vi "Autonomous Independent.vi"() -> ()   [LabVIEW 2019]
doc: "This VI is called when autonomous begins, and will automatically be terminated when autonomous ends. You can carry out timed or sensor driven robot movement independently without needing to return to the caller."
uses:
  <vilib>/Rock Robotics/WPI/ThirdParty/Phoenix-LabVIEW/Motor Controller/Controls/CTRE_Phoenix_MotorControl_ControlMode.ctl
  <vilib>/Rock Robotics/WPI/Utilities/WPI_GetSetVariantRefNum.vi
  <vilib>/Rock Robotics/Network Tables/NT Read String.vi
  <vilib>/Rock Robotics/Network Tables/NT Write Numeric Array.vi
  <vilib>/Rock Robotics/WPI/RobotDrive/WPI_RobotDriveArcadeDrive_Standard(NoSaturation).vi
panel:
  in  "Control Mode 4":T1 items=["PercentOutput"=0, "Position"=1, "Velocity"=2, "Current"=3, "Follower"=5, "MotionProfile"=6, "MotionMagic"=7, "MotionProfileArc"=10, "Disabled"=15]
  in  "Control Mode 3":T1 items=["PercentOutput"=0, "Position"=1, "Velocity"=2, "Current"=3, "Follower"=5, "MotionProfile"=6, "MotionMagic"=7, "MotionProfileArc"=10, "Disabled"=15]
  out "Current Movement, for debugging":T2 {"Y Joystick Value" scale=1.0..-1.0; "X Joystick Value" scale=-1.0..1.0}
  in  "Array of robot movements":T3(array[cluster])=[{"X Joystick Value"=0.39393939393939403, "Y Joystick Value"=0.0, "Delay (sec)"=1.0, "Movement Name"="turn"}, {"X Joystick Value"=-0.3737373737373737, "Y Joystick Value"=0.0, "Delay (sec)"=1.0, "Movement Name"="turn back"}] {"Y Joystick Value" scale=1.0..-1.0; "X Joystick Value" scale=-1.0..1.0}
  # "Be sure to right-click and choose Data Operations>>Make Current Value default if you want to save the array values with the VI"
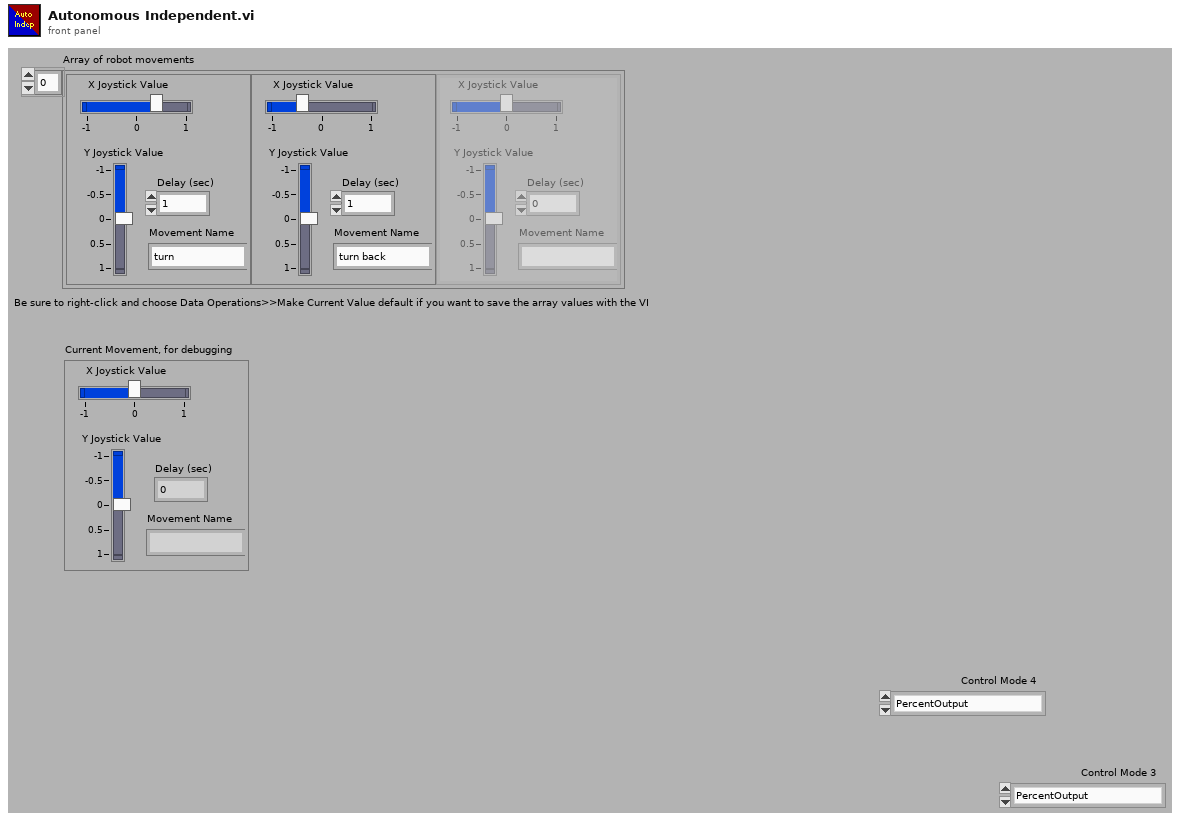
[diagram p1: front panel]
types:
  T1 = typedef "CTRE_Phoenix_MotorControl_ControlMode.ctl" = u16
  T2 = cluster{"X Joystick Value":dbl, "Y Joystick Value":dbl, "Delay (sec)":dbl, "Movement Name":string}
  T3 = cluster{"X Joystick Value":dbl, "Y Joystick Value":dbl, "Delay (sec)":dbl, "Movement Name":string}[]
  T4 = typedef "WPI_JoystickDevRef.ctl" = cluster{"Device":T5}
  T5 = typedef "WPI_JoystickDeviceEnum.ctl" = enum16{"USB 0", "USB 1", "USB 2", "USB 3", "USB 4", "USB 5"}
  T6 = typedef "WPI_RobotDriveDevRef.ctl" = cluster{"DevStatus":errorcluster, "Motors[]":T7[], "Square Inputs":bool, "Max Output":dbl}
  T7 = typedef "WPI_MotorControlDeviceRef.ctl" = cluster{"DeviceStatus":errorcluster, "Type":T8, "PWM":cluster{"PWM Channel":T9, "DeadBand":T10}, "CAN":cluster{"Device Number":u8, "SetOutput VI Ref":variant, "GetOutput VI Ref":variant, "Enable VI Ref":variant, "Disable VI Ref":variant, "Data":variant}, "Invert":bool, "DIO PWM":cluster{"PWM \"Enable\" Channel":T9, "DIOChannel":T11, "PWM Rate":dbl}}
  T8 = typedef "WPI_MotorControlType.ctl" = enum16{"PWM", "CAN", "DIO PWM"}
  T9 = typedef "FPGA_DIOPWMChannel.ctl" = enum8{"PWM 0", "PWM 1", "PWM 2", "PWM 3", "PWM 4", "PWM 5", "PWM 6", "PWM 7", "PWM 8", "PWM 9", "PWM MXP 0", "PWM MXP 1", "PWM MXP 2", "PWM MXP 3", "PWM MXP 4", "PWM MXP 5", "PWM MXP 6", "PWM MXP 7", "PWM MXP 8", "PWM MXP 9", "Invalid"}
  T10 = typedef "WPI_PWMDeadband.ctl" = cluster{"Name":string, "maxPositivePwm":i32, "minPositivePwm":i32, "centerPwm":i32, "maxNegativePwm":i32, "minNegativePwm":i32, "angularRange":u16}
  T11 = typedef "FPGA_DIOChannel.ctl" = enum8{"DIO 0", "DIO 1", "DIO 2", "DIO 3", "DIO 4", "DIO 5", "DIO 6", "DIO 7", "DIO 8", "DIO 9", "DIO MXP 0", "DIO MXP 1", "DIO MXP 2", "DIO MXP 3", "DIO MXP 4", "DIO MXP 5", "DIO MXP 6", "DIO MXP 7", "DIO MXP 8", "DIO MXP 9", "DIO MXP 10", "DIO MXP 11", "DIO MXP 12", "DIO MXP 13", "DIO MXP 14", "DIO MXP 15", "SPI Port CS1", "SPI Port CS2", "SPI Port CS3", "SPI Port MISO", "SPI Port MOSI", "Invalid"}
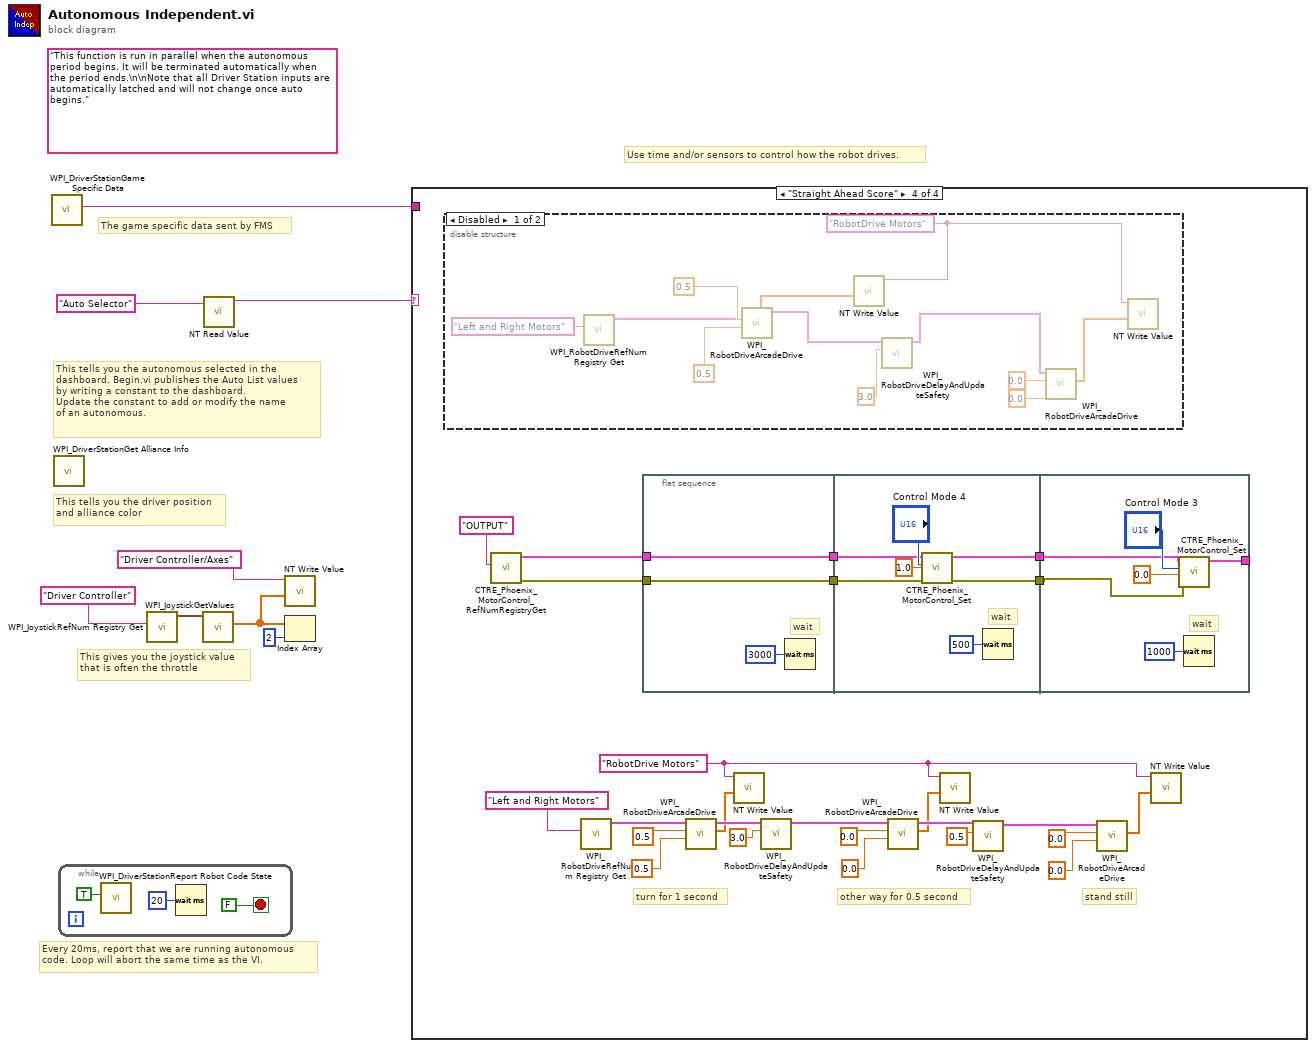
[diagram p0: block diagram]
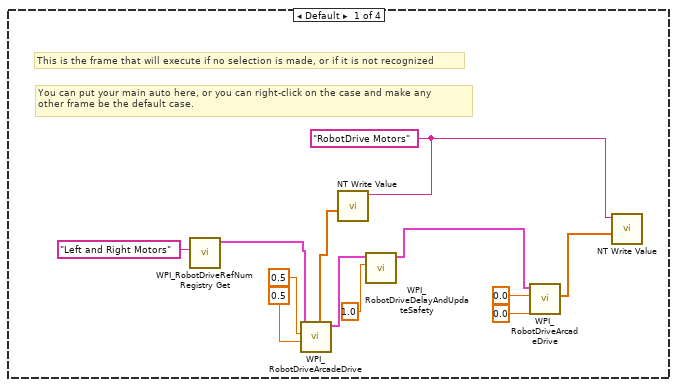
[diagram p2: hidden frame]
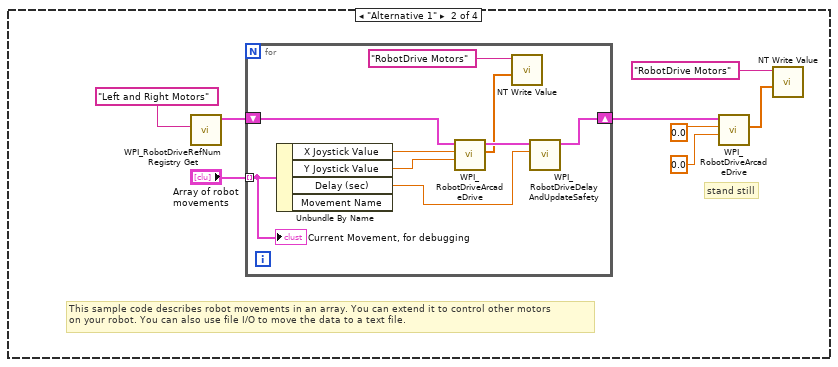
[diagram p3: hidden frame]
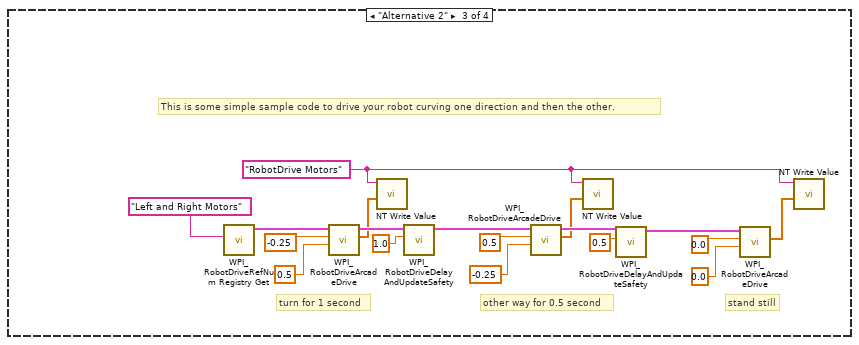
[diagram p4: hidden frame]
diagram:
  (unwired) "This function is run in parallel when the autonomous period begins. It will be terminated automatically when the period ends.\n\nNote that all Driver Station inputs are automatically latched and will not change once auto begins."
  # "The game specific data sent by FMS"
  # "This tells you the autonomous selected in the \ndashboard. Begin.vi publishes the Auto List values\nby writing a constant to the dashboard.\nUpdate the constant to add or modify the name\nof an autonomous."
  # "Every 20ms, report that we are running autonomous\ncode. Loop will abort the same time as the VI."
  # "This gives you the joystick value\nthat is often the throttle"
  # "Use time and/or sensors to control how the robot drives."
  # "This tells you the driver position\nand alliance color"
  n1 = call <vilib>:"WPI_DriverStationGame Specific Data.vi"() -> ("Game Specific Data"=w1:string)  [unwired: 11 in]
  n2 = call <vilib>:"WPI_DriverStationGet Alliance Info.vi"() -> ()  [unwired: 12 out]
  n3 = while {
    stop <- FALSE stop-if-true
    n4 = call <vilib>:"WPI_DriverStationReport Robot Code State.vi"("Autonomous"=TRUE) -> ()  [unwired: 10 in, 1 out]
    n5 = Wait (ms)(milliseconds to wait=u32 20) -> ()  [unwired: 1 out]
  }
  n6 = call <vilib>:"WPI_JoystickRefNum Registry Get.vi"("refnum name"="Driver Controller") -> ("JoystickDevRef"=w7:T4)  [unwired: 1 in, 9 out]
  n7 = call <vilib>:"WPI_JoystickGetValues.vi"("JoystickDevRef"=w7) -> ("Axes"=w3:dbl[])  [unwired: 6 in, 4 out]
  n8 = call-poly <vilib>:"NT Read Value.vi"("Name"="Auto Selector") -> ("String"=w4:string)  [unwired: 9 in, 1 out]
  n9 = call-poly <vilib>:"NT Write Value.vi"("Numeric Array"=w3, "Name"="Driver Controller/Axes") -> ()  [unwired: 9 in, 1 out]
  n10 = Index Array(array=w3, index=2) -> ()  [unwired: 1 out]
  n11 = case shown="\"Straight Ahead Score\"" w4 {
    tunnel: w1 -> [_ _ _ _]
    frame Default {
      w23 = "RobotDrive Motors" ("Name")
      # "You can put your main auto here, or you can right-click on the case and make any\nother frame be the default case."
      # "This is the frame that will execute if no selection is made, or if it is not recognized"
      n12 = call <vilib>:"WPI_RobotDriveRefNum Registry Get.vi"("refnum name"="Left and Right Motors") -> ("RobotDriveDevRef"=w19:T6)  [unwired: 9 in, 1 out]
      n13 = call-poly <vilib>:"WPI_RobotDriveArcadeDrive.vi"("Y axis value"=0.5, "X axis value"=0.5, "RobotDriveDevRef"=w19) -> ("Motor Values"=w17:dbl[], "RobotDriveDevRef"=w18:T6)  [unwired: 1 in, 6 out]
      n14 = call-poly <vilib>:"NT Write Value.vi"("Numeric Array"=w17, "Name"=w23) -> ()  [unwired: 9 in, 1 out]
      n15 = call <vilib>:"WPI_RobotDriveDelayAndUpdateSafety.vi"("Delay (s)"=1.0, "RobotDriveDevRef"=w18) -> ("RobotDriveDevRef 2"=w16:T6)  [unwired: 8 in, 1 out]
      n16 = call-poly <vilib>:"WPI_RobotDriveArcadeDrive.vi"("Y axis value"=0.0, "X axis value"=0.0, "RobotDriveDevRef"=w16) -> ("Motor Values"=w13:dbl[])  [unwired: 1 in, 7 out]
      n17 = call-poly <vilib>:"NT Write Value.vi"("Numeric Array"=w13, "Name"=w23) -> ()  [unwired: 9 in, 1 out]
    }
    frame "Alternative 1" {
      # "stand still"
      # "This sample code describes robot movements in an array. You can extend it to control other motors\non your robot. You can also use file I/O to move the data to a text file."
      n18 = call <vilib>:"WPI_RobotDriveRefNum Registry Get.vi"("refnum name"="Left and Right Motors") -> ("RobotDriveDevRef"=w30:T6)  [unwired: 1 in, 9 out]
      n19 = for {
        shift-right: [w38] -> w25
        shift-left: w30 -> [w39]
        tunnel: "Array of robot movements" -> [w34] mode=indexing
        n20 = Unbundle By Name(w34) -> ("X Joystick Value"=w37:dbl, "Y Joystick Value"=w36:dbl, "Delay (sec)"=w35:dbl)  [unwired: 1 out]
        n21 = call-poly <vilib>:"WPI_RobotDriveArcadeDrive.vi"("Y axis value"=w36, "X axis value"=w37, "RobotDriveDevRef"=w39) -> ("Motor Values"=w32:dbl[], "RobotDriveDevRef"=w40:T6)  [unwired: 1 in, 6 out]
        n22 = call-poly <vilib>:"NT Write Value.vi"("Numeric Array"=w32, "Name"="RobotDrive Motors") -> ()  [unwired: 9 in, 1 out]
        n23 = call <vilib>:"WPI_RobotDriveDelayAndUpdateSafety.vi"("Delay (s)"=w35, "RobotDriveDevRef"=w40) -> ("RobotDriveDevRef 2"=w38:T6)  [unwired: 8 in, 1 out]
        "Current Movement, for debugging" <- w34
      }
      n24 = call-poly <vilib>:"WPI_RobotDriveArcadeDrive.vi"("Y axis value"=0.0 ("X axis value"), "X axis value"=0.0, "RobotDriveDevRef"=w25) -> ("Motor Values"=w28:dbl[])  [unwired: 1 in, 7 out]
      n25 = call-poly <vilib>:"NT Write Value.vi"("Numeric Array"=w28, "Name"="RobotDrive Motors") -> ()  [unwired: 9 in, 1 out]
    }
    frame "Alternative 2" {
      w42 = "RobotDrive Motors" ("Name")
      # "This is some simple sample code to drive your robot curving one direction and then the other."
      # "stand still"
      # "other way for 0.5 second"
      # "turn for 1 second"
      n26 = call <vilib>:"WPI_RobotDriveRefNum Registry Get.vi"("refnum name"="Left and Right Motors") -> ("RobotDriveDevRef"=w58:T6)  [unwired: 1 in, 9 out]
      n27 = call-poly <vilib>:"WPI_RobotDriveArcadeDrive.vi"("Y axis value"=0.5 ("X axis value"), "X axis value"=-0.25, "RobotDriveDevRef"=w58) -> ("Motor Values"=w41:dbl[], "RobotDriveDevRef"=w51:T6)  [unwired: 1 in, 6 out]
      n28 = call-poly <vilib>:"NT Write Value.vi"("Numeric Array"=w41, "Name"=w42) -> ()  [unwired: 9 in, 1 out]
      n29 = call <vilib>:"WPI_RobotDriveDelayAndUpdateSafety.vi"("Delay (s)"=1.0, "RobotDriveDevRef"=w51) -> ("RobotDriveDevRef 2"=w52:T6)  [unwired: 8 in, 1 out]
      n30 = call-poly <vilib>:"WPI_RobotDriveArcadeDrive.vi"("Y axis value"=-0.25 ("X axis value"), "X axis value"=0.5, "RobotDriveDevRef"=w52) -> ("Motor Values"=w43:dbl[], "RobotDriveDevRef"=w53:T6)  [unwired: 1 in, 6 out]
      n31 = call-poly <vilib>:"NT Write Value.vi"("Numeric Array"=w43, "Name"=w42) -> ()  [unwired: 9 in, 1 out]
      n32 = call <vilib>:"WPI_RobotDriveDelayAndUpdateSafety.vi"("Delay (s)"=0.5, "RobotDriveDevRef"=w53) -> ("RobotDriveDevRef 2"=w54:T6)  [unwired: 8 in, 1 out]
      n33 = call-poly <vilib>:"WPI_RobotDriveArcadeDrive.vi"("Y axis value"=0.0 ("X axis value"), "X axis value"=0.0, "RobotDriveDevRef"=w54) -> ("Motor Values"=w44:dbl[])  [unwired: 1 in, 7 out]
      n34 = call-poly <vilib>:"NT Write Value.vi"("Numeric Array"=w44, "Name"=w42) -> ()  [unwired: 9 in, 1 out]
    }
    frame "Straight Ahead Score" {
      w60 = "RobotDrive Motors" ("Name")
      # "stand still"
      # "other way for 0.5 second"
      # "turn for 1 second"
      n35 = disable-structure shown="Disabled" {
        frame Disabled {
          w95 = "RobotDrive Motors" ("Name")
          n36 = call <vilib>:"WPI_RobotDriveRefNum Registry Get.vi"("refnum name"="Left and Right Motors") -> ("RobotDriveDevRef"=w91:T6)  [unwired: 9 in, 1 out]
          n37 = call-poly <vilib>:"WPI_RobotDriveArcadeDrive.vi"("Y axis value"=0.5, "X axis value"=0.5, "RobotDriveDevRef"=w91) -> ("Motor Values"=w89:dbl[], "RobotDriveDevRef"=w90:T6)  [unwired: 1 in, 6 out]
          n38 = call-poly <vilib>:"NT Write Value.vi"("Numeric Array"=w89, "Name"=w95) -> ()  [unwired: 9 in, 1 out]
          n39 = call <vilib>:"WPI_RobotDriveDelayAndUpdateSafety.vi"("Delay (s)"=3.0, "RobotDriveDevRef"=w90) -> ("RobotDriveDevRef 2"=w88:T6)  [unwired: 8 in, 1 out]
          n40 = call-poly <vilib>:"WPI_RobotDriveArcadeDrive.vi"("Y axis value"=0.0, "X axis value"=0.0, "RobotDriveDevRef"=w88) -> ("Motor Values"=w85:dbl[])  [unwired: 1 in, 7 out]
          n41 = call-poly <vilib>:"NT Write Value.vi"("Numeric Array"=w85, "Name"=w95) -> ()  [unwired: 9 in, 1 out]
        }
        frame Enabled {
        }
      }
      n42 = call <vilib>:"CTRE_Phoenix_MotorControl_RefNumRegistryGet.vi"("refnum name"="OUTPUT") -> ("error out"=w80:errorcluster, "PhoenixMotorControlDevRef"=w79:T7)  [unwired: 9 in]
      n43 = call <vilib>:"WPI_RobotDriveRefNum Registry Get.vi"("refnum name"="Left and Right Motors") -> ("RobotDriveDevRef"=w76:T6)  [unwired: 1 in, 9 out]
      n44 = flat-sequence {
        tunnel: w79 -> [w96]
        tunnel: [w97] -> w81
        tunnel: w80 -> [w97]
        tunnel: [w96] -> w77
        tunnel: [w99] -> w82
        tunnel: w81 -> [w100]
        tunnel: [w101] -> w78
        tunnel: w77 -> [w102]
        tunnel: w82 -> [w109]
        tunnel: w78 -> [w108]
        tunnel: [w106] -> _
        frame #0 {
          # "wait"
          n45 = Wait (ms)(milliseconds to wait=u32 3000) -> ()  [unwired: 1 out]
        }
        frame #1 {
          # "wait"
          n46 = call <vilib>:"CTRE_Phoenix_MotorControl_Set.vi"("error in (no error)"=w100, "Output"=1.0, "Control Mode"="Control Mode 4", "PhoenixMotorControlDevRef"=w102) -> ("error out"=w99:errorcluster, "PhoenixMotorControlDevRef"=w101:T7)  [unwired: 6 in]
          n47 = Wait (ms)(milliseconds to wait=u32 500) -> ()  [unwired: 1 out]
        }
        frame #2 {
          # "wait"
          n48 = call <vilib>:"CTRE_Phoenix_MotorControl_Set.vi"("error in (no error)"=w109, "Output"=0.0, "Control Mode"="Control Mode 3", "PhoenixMotorControlDevRef"=w108) -> ("PhoenixMotorControlDevRef"=w106:T7)  [unwired: 6 in, 1 out]
          n49 = Wait (ms)(milliseconds to wait=u32 1000) -> ()  [unwired: 1 out]
        }
      }
      n50 = call-poly <vilib>:"WPI_RobotDriveArcadeDrive.vi"("Y axis value"=0.5 ("X axis value"), "X axis value"=0.5, "RobotDriveDevRef"=w76) -> ("Motor Values"=w59:dbl[], "RobotDriveDevRef"=w69:T6)  [unwired: 1 in, 6 out]
      n51 = call-poly <vilib>:"NT Write Value.vi"("Numeric Array"=w59, "Name"=w60) -> ()  [unwired: 9 in, 1 out]
      n52 = call <vilib>:"WPI_RobotDriveDelayAndUpdateSafety.vi"("Delay (s)"=3.0, "RobotDriveDevRef"=w69) -> ("RobotDriveDevRef 2"=w70:T6)  [unwired: 8 in, 1 out]
      n53 = call-poly <vilib>:"WPI_RobotDriveArcadeDrive.vi"("Y axis value"=0.0 ("X axis value"), "X axis value"=0.0, "RobotDriveDevRef"=w70) -> ("Motor Values"=w61:dbl[], "RobotDriveDevRef"=w71:T6)  [unwired: 1 in, 6 out]
      n54 = call-poly <vilib>:"NT Write Value.vi"("Numeric Array"=w61, "Name"=w60) -> ()  [unwired: 9 in, 1 out]
      n55 = call <vilib>:"WPI_RobotDriveDelayAndUpdateSafety.vi"("Delay (s)"=0.5, "RobotDriveDevRef"=w71) -> ("RobotDriveDevRef 2"=w72:T6)  [unwired: 8 in, 1 out]
      n56 = call-poly <vilib>:"WPI_RobotDriveArcadeDrive.vi"("Y axis value"=0.0 ("X axis value"), "X axis value"=0.0, "RobotDriveDevRef"=w72) -> ("Motor Values"=w62:dbl[])  [unwired: 1 in, 7 out]
      n57 = call-poly <vilib>:"NT Write Value.vi"("Numeric Array"=w62, "Name"=w60) -> ()  [unwired: 9 in, 1 out]
    }
  }
